vi "SetParamPan.vi"(8 "error in (no error)":errorcluster caption="entrée d'erreur (pas d'erreur)", 11 "AppliedMotionDrive.lvclass":refnum<class "AppliedMotionDrive.lvclass">) -> (0 "error out":errorcluster caption="sortie d'erreur", 3 "AppliedMotionDrive.lvclass Out":refnum<class "AppliedMotionDrive.lvclass">)   [LabVIEW 2019, in "AppliedMotionDrive.lvclass"]
uses:
  AppliedMotionDrive.lvclass
  C:/Programmes Labview/LabscanV1A/DevicesClass/BaseDevice/BaseDevice.lvclass
panel:
  in  "Save  2":bool
  in  "Origine":bool
  in  "Nom":string
  in  "Save  2":bool
  in  "Save":bool
  in  "Accél Max":dbl=0.167 caption="Accélération Max \n(Tour/s/s)" min=0.167 max=5461.167 step=0.167 format="%#.3g"
  in  "Décél":dbl=0.167 caption="Décélération \n(Tour/s/s)" min=0.167 max=5461.167 step=0.167 format="%#.3g"
  in  "Accél":dbl=0.167 caption="Accélération \n(Tour/s/s)" min=0.167 max=5461.167 step=0.167 format="%#.3g"
  in  "Vitesse":dbl=0.08399999999999999 caption="Vitesse \n(Tour/s)" min=0.0042 max=133.3333 step=0.0042 format="%#.4g"
  out "CCW Limit":bool
  out "CW Limit":bool
  in  "Stop Move":bool
  in  "Stop":bool
  out "Init Program":bool
  # "Applied Motion Drive Parameters Panel"
  # "Paramètres du moteur"
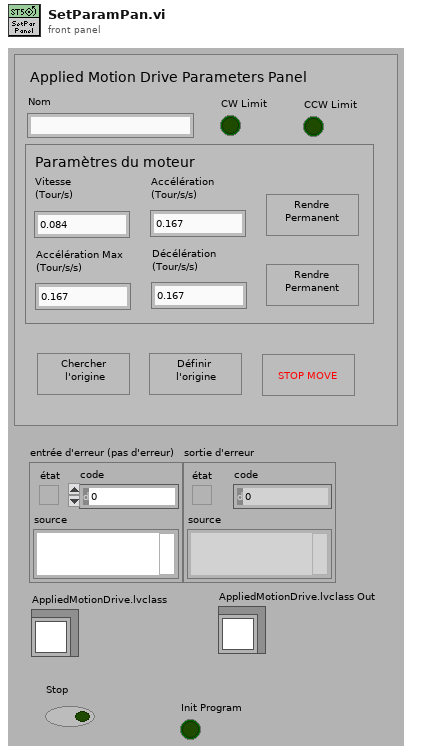
[diagram p1: front panel]
types:
  T1 = cluster{"Vitesse (Tour/s)":dbl, "Accél":dbl, "Décél":dbl, "Accél Max":dbl, "Idle Current (A) ":dbl}
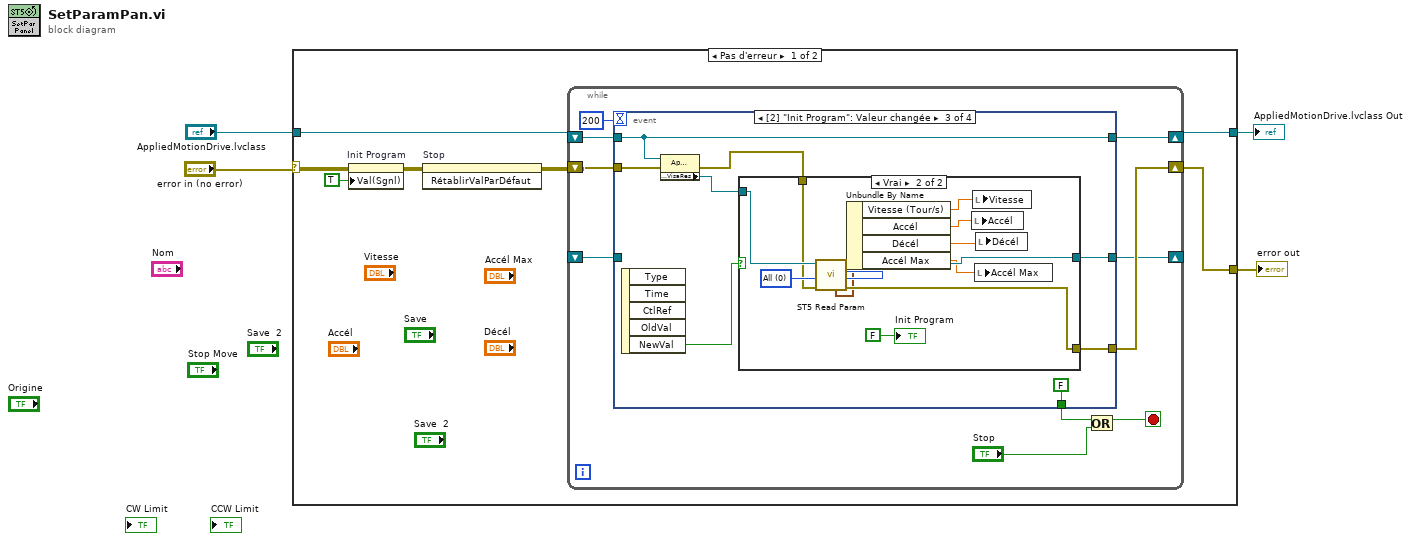
[diagram p0: block diagram]
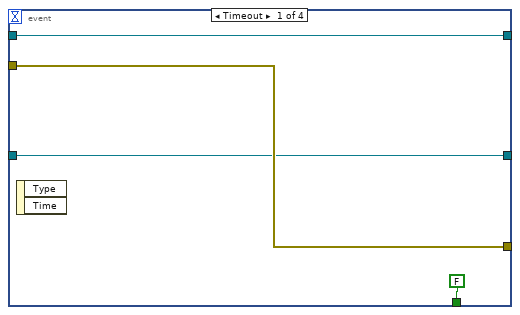
[diagram p2: hidden frame]
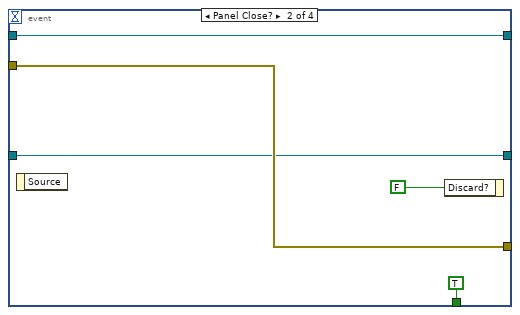
[diagram p3: hidden frame]
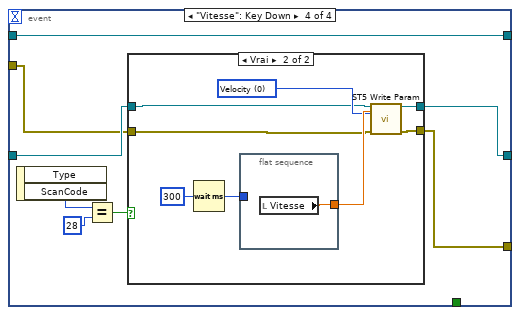
[diagram p5: hidden frame]
diagram:
  n1 = case shown="Pas d'erreur" "error in (no error)" {
    selector: "error in (no error)" -> [w8 w72]
    tunnel: [w11 w72] -> w3
    tunnel: "AppliedMotionDrive.lvclass" -> [w5 w71]
    tunnel: [w9 w71] -> w1
    frame No Error {
      n2 = property on="Init Program" class="Bool (strict)"(error in=w8, "Val(Sgnl)"=TRUE ("Valeur (Signalisation)")) -> (error out=w7:errorcluster)  [unwired: 1 in, 1 out]
      n3 = invoke on="Stop" class="Bool (strict)" method="RétablirValParDéfaut"(error in=w7) -> (error out=w6:errorcluster)  [unwired: 2 in, 2 out]
      n4 = while {
        shift-right: [w19] -> w11
        shift-left: w6 -> [w20]
        shift-right: [w16] -> w9
        shift-left: w5 -> [w18]
        shift-right: [w13] -> _
        shift-left: _ -> [w12]
        stop <- w15 stop-if-true
        n5 = event shown="[2] \"Init Program\": Valeur changée" {
          selector: _ -> [_ _ _ _]
          dyn-events: _ -> [_ _ _ _]
          timeout: 200 -> [_ _ _ _]
          tunnel: w20 -> [w23 w28 w35 w58]
          tunnel: [w23 w28 w37 w57] -> w19
          tunnel: w18 -> [w24 w27 w33 w52]
          tunnel: [FALSE TRUE FALSE _] -> w17
          tunnel: [w24 w27 w33 w52] -> w16
          tunnel: [w22 w26 w31 w56] -> w13
          tunnel: w12 -> [w22 w26 _ w59]
          event Timeout {
            n6 = event-data() -> ()  [unwired: 1 in, 2 out]
          }
          event Panel Close? {
            n7 = event-data() -> ()  [unwired: 1 in, 1 out]
            n8 = event-data("Discard?"=FALSE ("Rejeter ?")) -> ()  [unwired: 1 in, 1 out]
          }
          event "Init Program": Value Change {
            n9 = event-data() -> ("NewVal"=w38:bool)  [unwired: 1 in, 4 out]
            n10 = property class="AppliedMotionDrive.lvclass"(reference=w33, error in=w35) -> (error out=w34:errorcluster, "Accessor:VisaRes"=w32:refnum<visa-resource-name>)  [unwired: 1 out]
            n11 = case shown="Vrai" w38 {
              tunnel: w34 -> [w40 w47]
              tunnel: [w40 w46] -> w37
              tunnel: w32 -> [w39 w49]
              tunnel: [w39 w48] -> w31
              frame False {
              }
              frame True {
                w50 = u16 0 items=["All", "Velocity", "Acceleration", "Deceleration", "Max Acceleration", "Position"] ("Parameters")
                n12 = call <userlib>:"ST5 Read Param.vi"("error in (no error)"=w47, "Parameters"=w50, "Port COM"=w49) -> ("error out"=w46:errorcluster, "Port COM Out"=w48:refnum<visa-resource-name>, "Speed Par"=w45:T1)  [unwired: 2 in, 4 out]
                n13 = Unbundle By Name(w45) -> ("Vitesse (Tour/s)"=w44:dbl, "Accél"=w43:dbl, "Décél"=w42:dbl, "Accél Max"=w41:dbl)
                n14 = local write "Accél"(w43) -> ()
                n15 = local write "Vitesse"(w44) -> ()
                n16 = local write "Accél Max"(w41) -> ()
                n17 = local write "Décél"(w42) -> ()
                "Init Program" <- FALSE
              }
            }
          }
          event "Vitesse": Key Down {
            n18 = event-data() -> ("ScanCode"=w54:i16)  [unwired: 1 in, 1 out]
            n19 = Equal?(x=w54, y=i16 28) -> (x = y?=w53:bool)
            n20 = case shown="Vrai" w53 {
              tunnel: w59 -> [w60 w64]
              tunnel: w58 -> [w61 w65]
              tunnel: [w61 w69] -> w57
              tunnel: [w60 w62] -> w56
              frame False {
              }
              frame True {
                w67 = u16 0 items=["Velocity", "Acceleration", "Deceleration", "Max Acceleration", "Zero", "Save"] ("Parameters")
                n21 = Wait (ms)(milliseconds to wait=u32 300 ("attente (ms)")) -> (millisecond timer value=w63:u32)
                n22 = flat-sequence {
                  tunnel: [w70] -> w68
                  tunnel: w63 -> [_]
                  frame #0 {
                    n23 = local read "Vitesse"() -> (w70:dbl)
                  }
                }
                n24 = call <userlib>:"ST5 Write Param.vi"("Port COM"=w64, "Vitesse"=w68, "Parameters"=w67, "error in (no error)"=w65) -> ("Port COM Out"=w62:refnum<visa-resource-name>, "error out"=w69:errorcluster)  [unwired: 10 in]
              }
            }
          }
        }
        n25 = Or(x=w17, y="Stop") -> (x .or. y?=w15:bool)
      }
    }
    frame Error {
    }
  }
  "error out" <- w3
  "AppliedMotionDrive.lvclass Out" <- w1
